vi "AH_SND.vi"(7 "Tries":i32=5, 8 "error in (no error)":errorcluster, 9 "CMD":string, 10 "Data Cluster In":T1 {"GUI Data Cluster"."SBR" format="%08b"}, 11 "Config Cluster In":T3={"General"={"Config.ini"=path "", "Default Logging Path"=path ""}, "Hardware"={"Global T VAR"="", "Global B VAR"="", "VISAS"={"GEN COM"="", "SCOPE COM"="", "VNA COM"=""}, "Connected?"={"SCOPE"=FALSE, "GEN"=FALSE, "VNA"=FALSE}}, "Operation"={"Operation Mode"=enum."Logging", "Status"="", "NewLog?"=FALSE, "OvenWarn"=FALSE, "Scope Settings"={"TimeBase"=0.0, "VerticalScale"=4.0}}}) -> (0 "error IO":errorcluster, 2 "Data Cluster Out":T1 {"GUI Data Cluster"."SBR" format="%08b"}, 3 "Configuration Cluster Out":T3={"General"={"Config.ini"=path "", "Default Logging Path"=path ""}, "Hardware"={"Global T VAR"="", "Global B VAR"="", "VISAS"={"GEN COM"="", "SCOPE COM"="", "VNA COM"=""}, "Connected?"={"SCOPE"=FALSE, "GEN"=FALSE, "VNA"=FALSE}}, "Operation"={"Operation Mode"=enum."Idle-Off", "Status"="", "NewLog?"=FALSE, "OvenWarn"=FALSE, "Scope Settings"={"TimeBase"=0.0, "VerticalScale"=4.0}}})   [LabVIEW 2021]
uses:
  Status_Byte.ctl
  Mode_Enum.ctl
  Config_Cluster.ctl
  Measurement_Cluster.ctl
  Data_Cluster.ctl
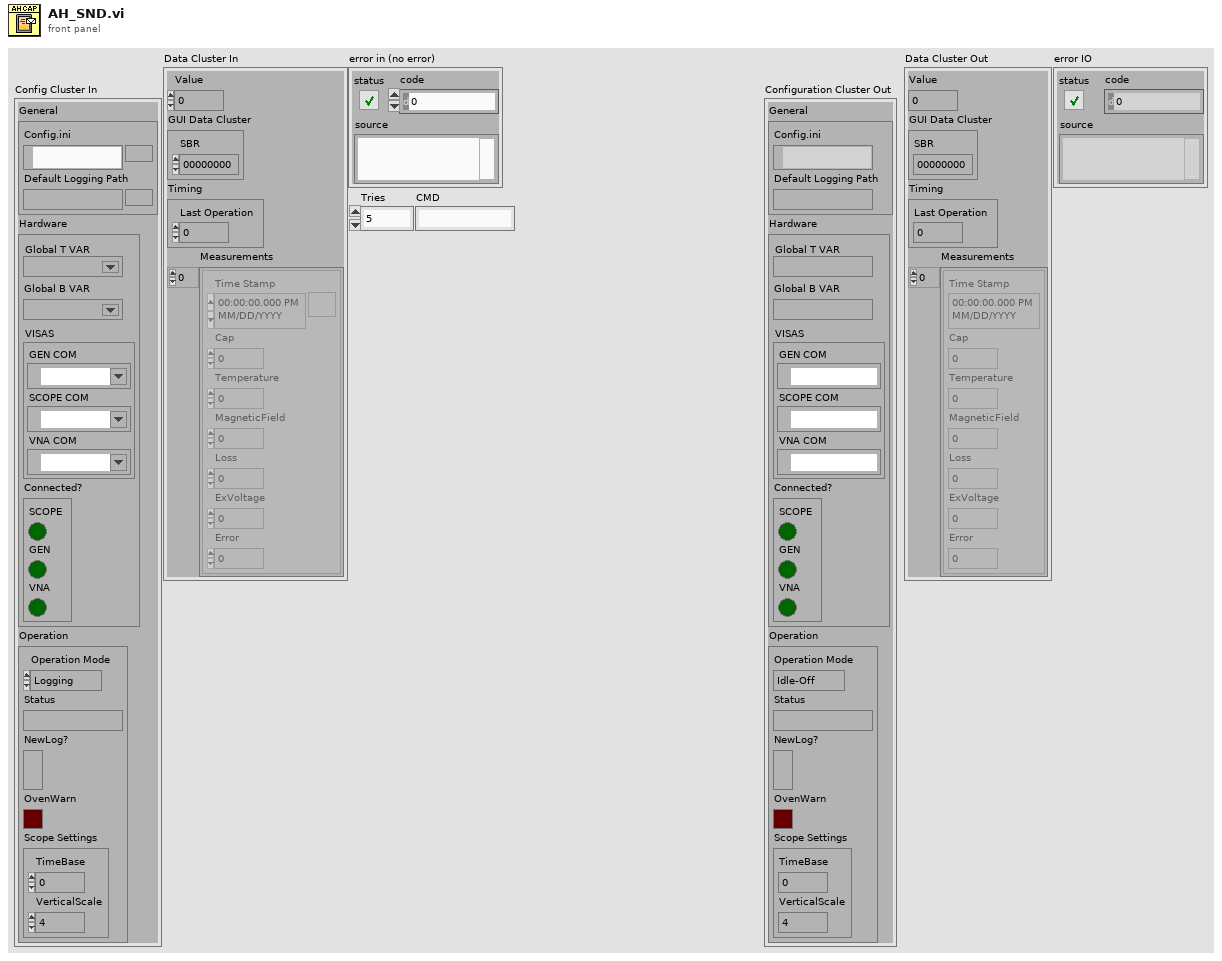
[diagram p1: front panel]
types:
  T1 = typedef "Data_Cluster.ctl" = cluster{"Value":dbl, "GUI Data Cluster":cluster{"SBR":u16}, "Timing":cluster{"Last Operation":dbl}, "Measurements":T2[]}
  T2 = typedef "Measurement_Cluster.ctl" = cluster{"Time Stamp":timestamp, "Cap":dbl, "Temperature":dbl, "MagneticField":dbl, "Loss":dbl, "ExVoltage":dbl, "Error":dbl}
  T3 = typedef "Config_Cluster.ctl" = cluster{"General":cluster{"Config.ini":path, "Default Logging Path":path}, "Hardware":cluster{"Global T VAR":refnum<k21>, "Global B VAR":refnum<k21>, "VISAS":cluster{"GEN COM":refnum<visa-resource-name>, "SCOPE COM":refnum<visa-resource-name>, "VNA COM":refnum<visa-resource-name>}, "Connected?":cluster{"SCOPE":bool, "GEN":bool, "VNA":bool}}, "Operation":cluster{"Operation Mode":T4, "Status":string, "NewLog?":bool, "OvenWarn":bool, "Scope Settings":cluster{"TimeBase":dbl, "VerticalScale":dbl}}}
  T4 = typedef "Mode_Enum.ctl" = enum16{"OvenNRDY", "Logging", "Idle-Off", "Idle"}
  T5 = typedef "Status_Byte.ctl" = u16
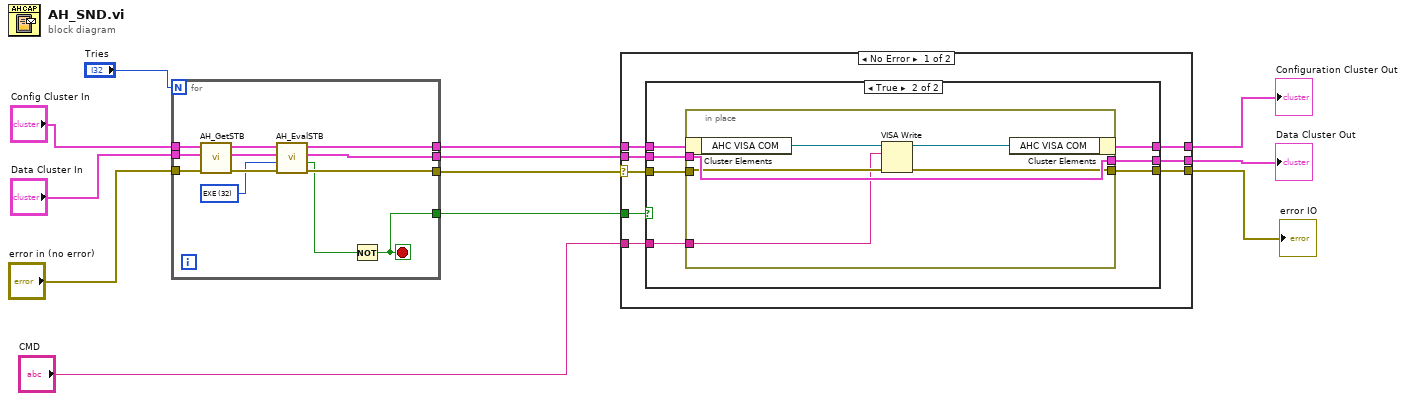
[diagram p0: block diagram]
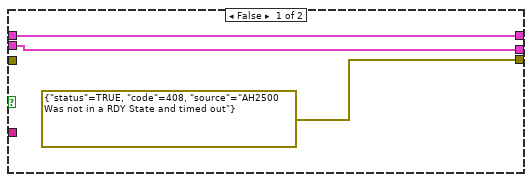
[diagram p2: hidden frame]
diagram:
  n1 = for {
    N: "Tries" -> [_]
    tunnel: "Config Cluster In" -> [w24]
    tunnel: "Data Cluster In" -> [w22]
    tunnel: "error in (no error)" -> [w21]
    tunnel: [w17] -> w7
    tunnel: [w16] -> w6
    tunnel: [w15] -> w8
    tunnel: [w14] -> w1
    stop <- w14 stop-if-true
    w18 = T5 32 items=["ONR"=1, "CME"=2, "URQ"=4, "PON"=8, "RDY"=16, "EXE"=32, "RQS"=64, "MAV"=128] ("Status Byte")
    n2 = call "AH_GetSTB.vi"("error in (no error)"=w21, "Data Cluster In"=w22, "Config Cluster In"=w24) -> ("error out"=w19:errorcluster, "Data Cluster Out"=w20:T1, "Configuration Cluster Out"=w23:T3)  [unwired: 6 in]
    n3 = call "AH_EvalSTB.vi"("error in (no error)"=w19, "Status Byte"=w18, "Data Cluster In"=w20, "Config Cluster In"=w23) -> ("error out"=w15:errorcluster, "Result"=w13:bool, "Data Cluster Out"=w16:T1, "Configuration Cluster Out"=w17:T3)  [unwired: 3 in, 1 out]
    n4 = Not(x=w13) -> (.not. x?=w14:bool)
  }
  n5 = case shown="No Error" w8 {
    selector: w8 -> [w29 w49]
    tunnel: w7 -> [w31 w51]
    tunnel: w6 -> [w30 w50]
    tunnel: w1 -> [w32 _]
    tunnel: [w28 w51] -> w4
    tunnel: [w27 w50] -> w3
    tunnel: [w26 w49] -> w2
    tunnel: "CMD" -> [w25 _]
    frame No Error {
      n6 = case shown="True" w32 {
        tunnel: w31 -> [w35 w42]
        tunnel: w30 -> [w34 w41]
        tunnel: w29 -> [_ w40]
        tunnel: [w35 w39] -> w28
        tunnel: [w34 w38] -> w27
        tunnel: [errorcluster {"status"=TRUE, "code"=408, "source"="AH2500 Was not in a RDY State and timed out"} ("error out") w37] -> w26
        tunnel: w25 -> [_ w36]
        frame False {
        }
        frame True {
          n7 = in-place {
            in-place-border: w41 -> [w46]
            in-place-border: w40 -> [w45]
            in-place-border: [w46] -> w38
            in-place-border: [w44] -> w37
            in-place-border: w36 -> [w43]
            n8 = in-place-cluster #1(w42) -> ("AHC VISA COM"=w48:refnum<visa-resource-name>)
            n9 = VISA Write(VISA resource name=w48, write buffer=w43, error in (no error)=w45) -> (VISA resource name out=w47:refnum<visa-resource-name>, error out=w44:errorcluster)  [unwired: 1 out]
            n10 = in-place-cluster #1("AHC VISA COM"=w47) -> (w39:T3)
          }
        }
      }
    }
    frame Error {
    }
  }
  "Configuration Cluster Out" <- w4
  "Data Cluster Out" <- w3
  "error IO" <- w2
